vi "Build LF Tasks.vi"(8 "error in":errorcluster, 11 "CRDS in":refnum<class "CRDS.lvclass">=refnum) -> (0 "error out":errorcluster, 3 "CRDS out":refnum<class "CRDS.lvclass">)   [LabVIEW 2012, in "CRDS.lvclass"]
doc: "This VI configures the low frequency signals on the M-series card. The appropriate configuration file entries are first read in. The scales for the AI signals are then setup. The scales are:\n\n* RHw = 20*Vin (0 to 100%)\n* Trh = 20*Vin - 40 (-40degC to 60degC)\n* P = 3*PSI->mb*Vin (0 to 15 psi)\n* T = uses the Steihart-Hart equations to take the Vin and covnert to a temperature for the appropriate thermistor constants\n\nAfter the scales are setup, the tasks are built by adding channels described in the config channel using the appropriate limits and scales. Each channel will be named using the measurement type (mType) and the cell number (Cell). The names will be something like T_1 for pressure measurements on cell 1. The low frequency signals are acquired at the rate fhkAI.\n\nIn addition, the tasks controlling the valves and acquiring the valves positions are setup."
uses:
  CRDS.lvclass
  Controls/Configuration/CRD Cell Num.ctl
  Controls/Configuration/LFConfig.ctl
  PAS_CRDS new/CRDS/Controls/LF_AI Clstr.ctl
  <vilib>/DAQmx/create/channels.llb/DAQmx Create Channel (AI-Voltage-Basic).vi
  <vilib>/DAQmx/configure/timing.llb/DAQmx Timing (Sample Clock).vi
  General/Atmospheric/Atmospheric Constants.vi
  General/Atmospheric/Atmospheric Library.lvlib
  <vilib>/DAQmx/create/channels.llb/DAQmx Create Channel (DI-Digital Input).vi
  Controls/Configuration/DIO Control.ctl
  <vilib>/DAQmx/create/channels.llb/DAQmx Create Channel (DO-Digital Output).vi
  Data Class/Main Class/CRDS Data.lvclass
  Controls/Configuration/mType.ctl
  <vilib>/Utility/config.llb/NI_LVConfig.lvlib
  <vilib>/Utility/config.llb/Read Key (String).vi
  <resource>/objmgr/daqmx.rc
  <vilib>/Utility/config.llb/Config Data RefNum.ctl
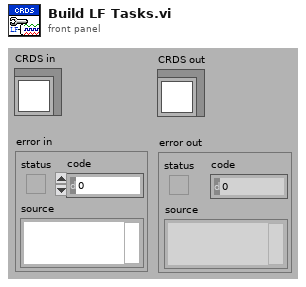
[diagram p1: front panel]
types:
  T1 = typedef "NI_LVConfig.lvlib/Config Data RefNum.ctl" = refnum<k1>
  T2 = typedef "DIO Control.ctl" = cluster{"DAQmx Physical Channel":tag, "Instrument":enum16{"CRDS", "PAS"}}[]
  T3 = typedef "LF_AI Clstr.ctl" = T4[]
  T4 = typedef "LFConfig.ctl" = cluster{"Name":string, "dmxCh":tag, "Cell":T5, "mType":T6, "Enable":bool}
  T5 = typedef "CRD Cell Num.ctl" = enum16{"Cell 1", "Cell 2", "Cell 3", "Cell 4", "Cell 5", "Cell 6", "Cell 7", "Cell 8", "None"}
  T6 = typedef "mType.ctl" = enum16{"Trh", "P", "T1", "T2", "RHw", "UDF1", "UDF2", "UDF3"}
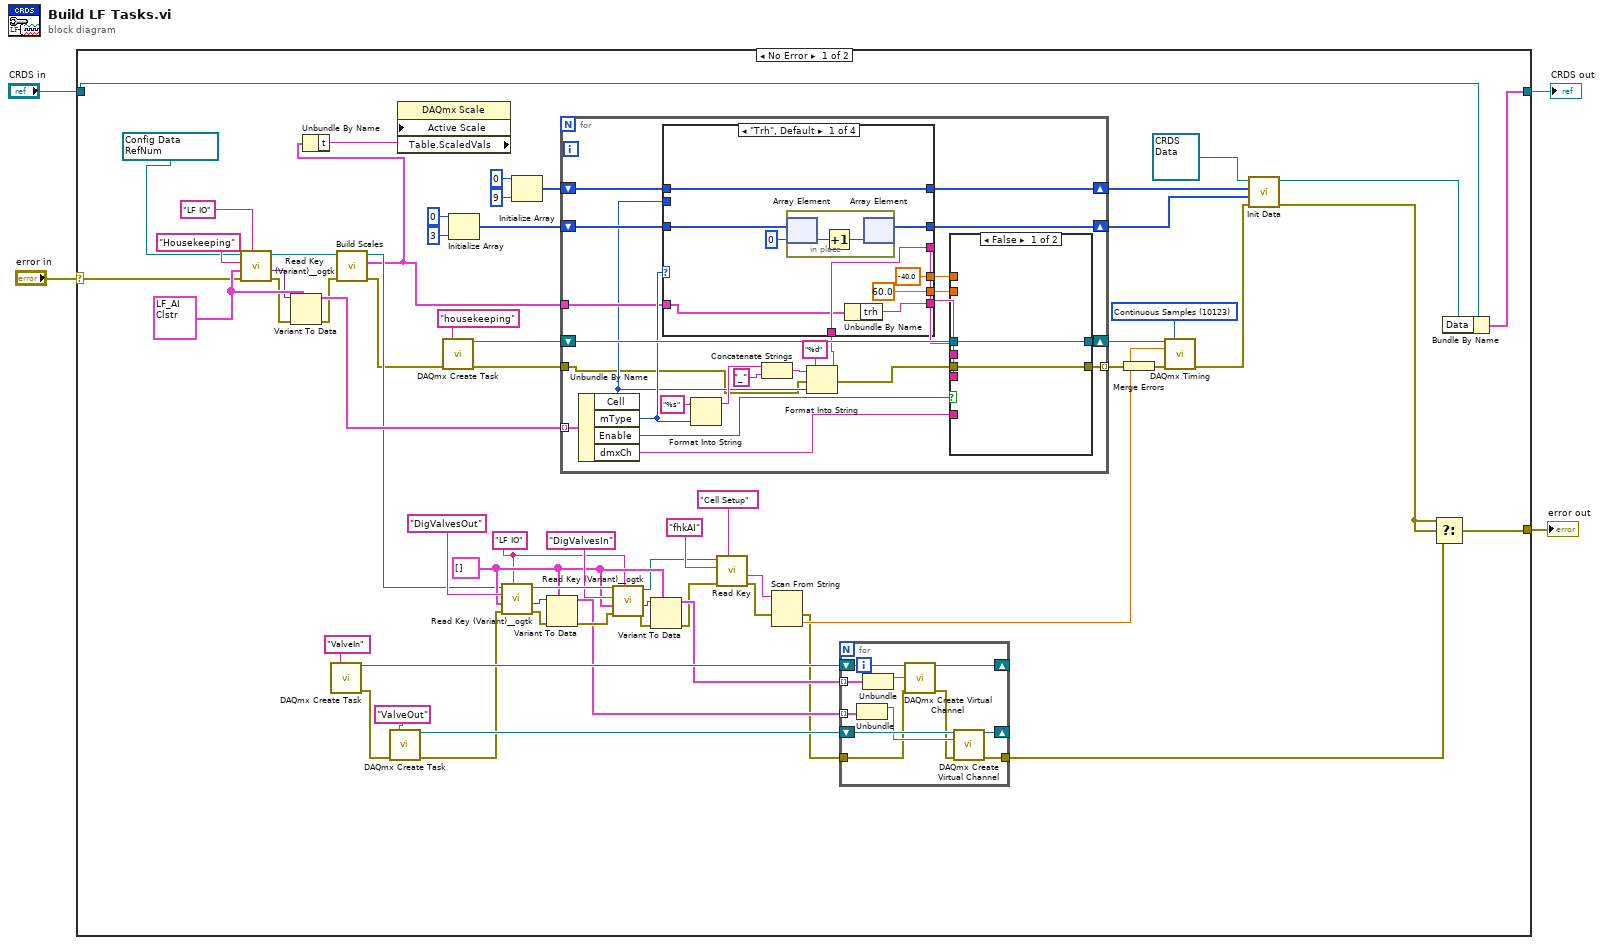
[diagram p0: block diagram]
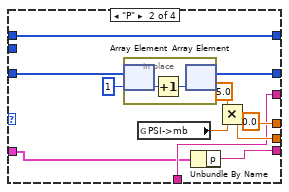
[diagram p2: hidden frame]
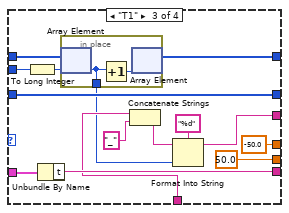
[diagram p3: hidden frame]
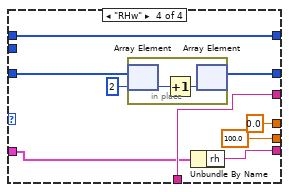
[diagram p4: hidden frame]
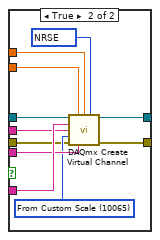
[diagram p5: hidden frame]
diagram:
  n1 = case shown="No Error" "error in" {
    selector: "error in" -> [w62 w170]
    tunnel: [w32 w170] -> w3
    tunnel: [w50 w169] -> w1
    tunnel: "CRDS in" -> [w51 w169]
    frame No Error {
      w5 = T1 refnum items=["config data"] ("refnum")
      w31 = "LF IO" ("section")
      w38 = T2 [] ("digValvesIn")
      w59 = 10123 items=["Finite Samples"=10178, "Continuous Samples"=10123, "Hardware Timed Single Point"=12522] ("sample mode")
      w67 = T3 [{"Name"="", "dmxCh"="", "Cell"=enum."Cell 1", "mType"=enum."Trh", "Enable"=FALSE}, {"Name"="", "dmxCh"="", "Cell"=enum."Cell 1", "mType"=enum."Trh", "Enable"=FALSE}, {"Name"="", "dmxCh"="", "Cell"=enum."Cell 1", "mType"=enum."Trh", "Enable"=FALSE}, {"Name"="", "dmxCh"="", "Cell"=enum."Cell 1", "mType"=enum."Trh", "Enable"=FALSE}, {"Name"="", "dmxCh"="", "Cell"=enum."Cell 1", "mType"=enum."Trh", "Enable"=FALSE}, {"Name"="", "dmxCh"="", "Cell"=enum."Cell 1", "mType"=enum."Trh", "Enable"=FALSE}, {"Name"="", "dmxCh"="", "Cell"=enum."Cell 1", "mType"=enum."Trh", "Enable"=FALSE}, {"Name"="", "dmxCh"="", "Cell"=enum."Cell 1", "mType"=enum."Trh", "Enable"=FALSE}, {"Name"="", "dmxCh"="", "Cell"=enum."Cell 1", "mType"=enum."Trh", "Enable"=FALSE}, {"Name"="", "dmxCh"="", "Cell"=enum."Cell 1", "mType"=enum."Trh", "Enable"=FALSE}, {"Name"="", "dmxCh"="", "Cell"=enum."Cell 1", "mType"=enum."Trh", "Enable"=FALSE}, {"Name"="", "dmxCh"="", "Cell"=enum."Cell 1", "mType"=enum."Trh", "Enable"=FALSE}, {"Name"="", "dmxCh"="", "Cell"=enum."Cell 1", "mType"=enum."Trh", "Enable"=FALSE}, {"Name"="", "dmxCh"="", "Cell"=enum."Cell 1", "mType"=enum."Trh", "Enable"=FALSE}, {"Name"="", "dmxCh"="", "Cell"=enum."Cell 1", "mType"=enum."Trh", "Enable"=FALSE}, {"Name"="", "dmxCh"="", "Cell"=enum."Cell 1", "mType"=enum."Trh", "Enable"=FALSE}, {"Name"="", "dmxCh"="", "Cell"=enum."Cell 1", "mType"=enum."Trh", "Enable"=FALSE}, {"Name"="", "dmxCh"="", "Cell"=enum."Cell 1", "mType"=enum."Trh", "Enable"=FALSE}, {"Name"="", "dmxCh"="", "Cell"=enum."Cell 1", "mType"=enum."Trh", "Enable"=FALSE}, {"Name"="", "dmxCh"="", "Cell"=enum."Cell 1", "mType"=enum."Trh", "Enable"=FALSE}, {"Name"="", "dmxCh"="", "Cell"=enum."Cell 1", "mType"=enum."Trh", "Enable"=FALSE}] ("lfAICh")
      n2 = call <userlib>:"Read Key (Variant)__ogtk.vi"("section"="LF IO", "error in (no error)"=w62, "type"=w67, "key (optional)"="Housekeeping", "refnum"=w5) -> ("error out"=w64:errorcluster, "key-value"=w65:variant, "refnum out"=w16:T1)  [unwired: 3 in, 1 out]
      n3 = Variant To Data(error in=w64, type=w67, Variant=w65) -> (data=w57:T3, error out=w15:errorcluster)
      n4 = call <vilib>:"DAQmx Create Task.vi"("new task name"="ValveIn") -> ("task out"=w49:refnum<k21>, "error out"=w47:errorcluster)  [unwired: 13 in]
      n5 = call "Build Scales.vi"("error in"=w15, "cfgFileIn"=w16) -> ("error out"=w10:errorcluster, "Scales"=w7:cluster{"trh":tag, "p":tag, "t":tag, "rh":tag}, "cfgFileOut"=w18:T1)  [unwired: 7 in]
      n6 = Unbundle By Name(w7) -> ("t"=w6:tag)
      n7 = call <vilib>:"DAQmx Create Task.vi"("new task name"="ValveOut", "error in"=w47) -> ("task out"=w48:refnum<k21>, "error out"=w12:errorcluster)  [unwired: 12 in]
      n8 = property class="DAQmx Scale" props=["Active Scale", "Table.ScaledVals"]("Active Scale"=w6) -> ()  [unwired: 2 in, 3 out]
      n9 = call <vilib>:"DAQmx Create Task.vi"("new task name"="housekeeping", "error in"=w10) -> ("task out"=w61:refnum<k21>, "error out"=w60:errorcluster)  [unwired: 12 in]
      n10 = Initialize Array(0 ("element"), 3 ("dimension size")) -> (w28:i32[])
      n11 = call <userlib>:"Read Key (Variant)__ogtk.vi"("section"=w31, "error in (no error)"=w12, "type"=w38, "key (optional)"="DigValvesOut", "refnum"=w18) -> ("error out"=w42:errorcluster, "key-value"=w43:variant, "refnum out"=w45:T1)  [unwired: 3 in, 1 out]
      n12 = Initialize Array(0 ("element"), 9 ("dimension size")) -> (w23:i32[])
      n13 = Variant To Data(error in=w42, type=w38, Variant=w43) -> (data=w34:T2, error out=w41:errorcluster)
      n14 = for {
        tunnel: w57 -> [w100] mode=indexing
        shift-right: [w101] -> w58
        shift-left: w61 -> [w103]
        tunnel: w60 -> [w80]
        tunnel: [w102] -> w9 mode=indexing
        shift-right: [w87] -> w22
        shift-left: w28 -> [w88]
        shift-right: [w85] -> w21
        shift-left: w23 -> [w86]
        tunnel: w7 -> [w82]
        n15 = Unbundle By Name(w100) -> ("Cell"=w81:T5, "mType"=w94:T6, "Enable"=w98:bool, "dmxCh"=w99:tag)
        n16 = Format Into String(format string="%s", w94) -> (resulting string=w92:string)  [unwired: 2 in, 1 out]
        n17 = Concatenate Strings(w92, "_" ("string")) -> (w90:string)
        n18 = Format Into String(format string="%d", initial string=w90, error in=w80, w81) -> (resulting string=w84:string, error out=w79:errorcluster)
        n19 = case shown="\"Trh\", Default" w94 {
          tunnel: [w112 w125 w142 w153] -> w97
          tunnel: [-40.0 ("minimum value") 0.0 ("minimum value") -50.0 ("minimum value") 0.0 ("minimum value")] -> w96
          tunnel: [60.0 w122 50.0 100.0] -> w95
          tunnel: w88 -> [w109 w121 w137 w150]
          tunnel: [w108 w119 w137 w149] -> w87
          tunnel: w86 -> [w107 w118 w139 w148]
          tunnel: w81 -> [_ _ w135 _]
          tunnel: [w107 w118 w138 w148] -> w85
          tunnel: w84 -> [w106 w117 w134 w147]
          tunnel: [w106 w117 w129 w147] -> w83
          tunnel: w82 -> [w105 w116 w128 w146]
          frame "Trh", Default {
            n20 = in-place {
              n21 = in-place-array #1(w109, 0) -> (w114:i32)
              n22 = Increment(x=w114) -> (x+1=w113:i32)
              n23 = in-place-array #1(w113) -> (w108:i32[])  [unwired: 1 out]
            }
            n24 = Unbundle By Name(w105) -> ("trh"=w112:tag)
          }
          frame "P" {
            n25 = in-place {
              n26 = in-place-array #2(w121, 1) -> (w127:i32)
              n27 = Increment(x=w127) -> (x+1=w126:i32)
              n28 = in-place-array #2(w126) -> (w119:i32[])  [unwired: 1 out]
            }
            n29 = global read "Atmospheric Constants.vi" "PSI->mb"() -> (w123:sgl)
            n30 = Unbundle By Name(w116) -> ("p"=w125:tag)
            n31 = Multiply(x=5.0 ("slope"), y=w123) -> (x*y=w122:dbl)
          }
          frame "T1" {
            n32 = To Long Integer(number=w135) -> (32bit integer=w136:i32)
            n33 = Unbundle By Name(w128) -> ("t"=w142:tag)
            n34 = in-place {
              in-place-border: [w143] -> w130
              n35 = in-place-array #3(w139, w136) -> (w143:i32)
              n36 = Increment(x=w143) -> (x+1=w144:i32)
              n37 = in-place-array #3(w144) -> (w138:i32[])  [unwired: 1 out]
            }
            n38 = Concatenate Strings(w134, "_" ("string")) -> (w131:string)
            n39 = Format Into String(format string="%d", initial string=w131, w130) -> (resulting string=w129:string)  [unwired: 1 in, 1 out]
          }
          frame "RHw" {
            n40 = in-place {
              n41 = in-place-array #4(w150, 2) -> (w155:i32)
              n42 = Increment(x=w155) -> (x+1=w154:i32)
              n43 = in-place-array #4(w154) -> (w149:i32[])  [unwired: 1 out]
            }
            n44 = Unbundle By Name(w146) -> ("rh"=w153:tag)
          }
        }
        n45 = case shown="False" w98 {
          tunnel: w99 -> [_ w168]
          tunnel: w103 -> [w157 w167]
          tunnel: [w156 w166] -> w102
          tunnel: [w157 w165] -> w101
          tunnel: w97 -> [_ w163]
          tunnel: w96 -> [_ w162]
          tunnel: w95 -> [_ w161]
          tunnel: w83 -> [_ w160]
          tunnel: w79 -> [w156 w158]
          frame False {
          }
          frame True {
            w159 = 10065 items=["Volts"=10348, "From Custom Scale"=10065] ("units")
            w164 = 10078 items=["default"=-1, "RSE"=10083, "NRSE"=10078, "Differential"=10106, "Pseudodifferential"=12529] ("input terminal configuration")
            n46 = call-poly <vilib>:"DAQmx Create Virtual Channel.vi"("task in"=w167, "maximum value"=w161, "minimum value"=w162, "input terminal configuration"=w164, "physical channels"=w168, "name to assign"=w160, "units"=w159, "error in"=w158, "custom scale name"=w163) -> ("task out"=w165:refnum<k21>, "error out"=w166:errorcluster)  [unwired: 5 in]
          }
        }
      }
      n47 = call <userlib>:"Read Key (Variant)__ogtk.vi"("section"=w31, "error in (no error)"=w41, "type"=w38, "key (optional)"="DigValvesIn", "refnum"=w45) -> ("error out"=w39:errorcluster, "key-value"=w40:variant, "refnum out"=w14:T1)  [unwired: 3 in, 1 out]
      n48 = Variant To Data(error in=w39, type=w38, Variant=w40) -> (data=w35:T2, error out=w13:errorcluster)
      n49 = call-poly <vilib>:"Read Key.vi"("section"="Cell Setup", "error in (no error)"=w13, "key"="fhkAI", "refnum"=w14) -> ("error out"=w17:errorcluster, "value"=w53:string)  [unwired: 4 in, 2 out]
      n50 = Scan From String(input string=w53, error in=w17) -> (error out=w11:errorcluster, output 1=w52:dbl)  [unwired: 3 in, 2 out]
      n51 = for {
        tunnel: w35 -> [w72] mode=indexing
        tunnel: w34 -> [w77] mode=indexing
        tunnel: w11 -> [w69]
        tunnel: [w74] -> w33
        shift-right: [w75] -> _
        shift-left: w48 -> [w78]
        shift-right: [w70] -> _
        shift-left: w49 -> [w73]
        n52 = Unbundle(w77) -> ("DAQmx Physical Channel"=w76:tag)  [unwired: 1 out]
        n53 = Unbundle(w72) -> ("DAQmx Physical Channel"=w71:tag)  [unwired: 1 out]
        n54 = call-poly <vilib>:"DAQmx Create Virtual Channel.vi"("task in"=w73, "lines"=w71, "error in"=w69) -> ("task out"=w70:refnum<k21>, "error out"=w68:errorcluster)  [unwired: 11 in]
        n55 = call-poly <vilib>:"DAQmx Create Virtual Channel.vi"("task in"=w78, "lines"=w76, "error in"=w68) -> ("task out"=w75:refnum<k21>, "error out"=w74:errorcluster)  [unwired: 11 in]
      }
      n56 = Merge Errors(w9) -> (w8:errorcluster)
      n57 = call-poly <vilib>:"DAQmx Timing.vi"("task/channels in"=w58, "sample mode"=w59, "rate"=w52, "error in"=w8) -> ("error out"=w26:errorcluster)  [unwired: 3 in, 8 out]
      n58 = call "Init Data.vi"("error in"=w26, "NumElem"=w22, "NumTs"=w21, "CRDS Data in"=refnum<class "CRDS Data.lvclass"> refnum) -> ("error out"=w19:errorcluster, "CRDS Data out"=w20:refnum<class "CRDS Data.lvclass">)  [unwired: 6 in]
      n59 = Select(t=w19, s=w19, f=w33) -> (s? t:f=w32:errorcluster)
      n60 = Bundle By Name(cluster=w51, "Data"=w20) -> (w50:cluster{})
    }
    frame Error {
    }
  }
  "error out" <- w3
  "CRDS out" <- w1
